vi "PFI-28000-Chan-Bridge_Get Filter Cutoff.vi"(8 "error in (no error)":errorcluster, 11 "PFI-28000-Chan-Bridge in":refnum<class "PFI-28000-Chan-Bridge.lvclass">) -> (0 "error out":errorcluster, 2 "Filter Cutoff":dbl, 3 "PFI-28000-Chan-Bridge out":refnum<class "PFI-28000-Chan-Bridge.lvclass">)   [LabVIEW 2017, in "PFI-28000-Chan-Bridge.lvclass"]
uses:
  PFI-28000-Chan-Bridge.lvclass
  C:/wc/07143 Precision Filters 28000 Support/Driver/source/Channel/PFI-28000-Channel.lvclass
  Utilities/PFI-28000-Utils.lvlib
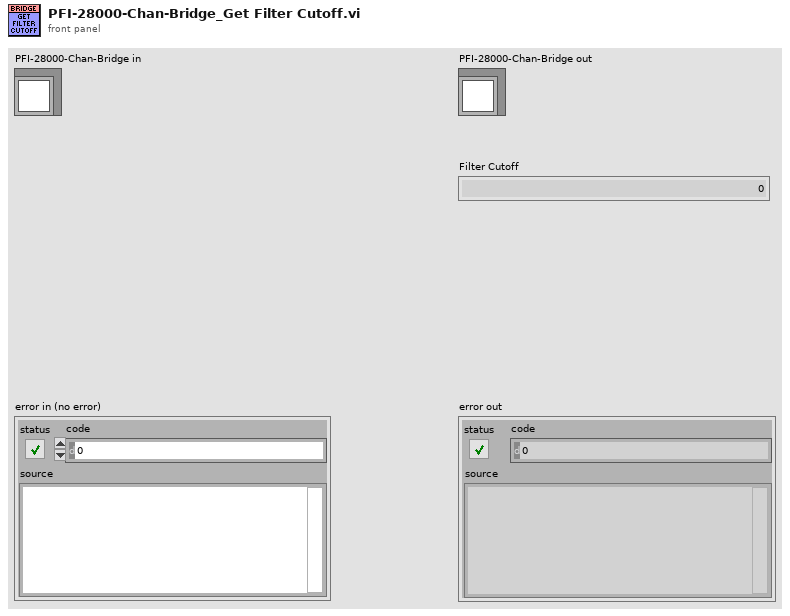
[diagram p1: front panel]
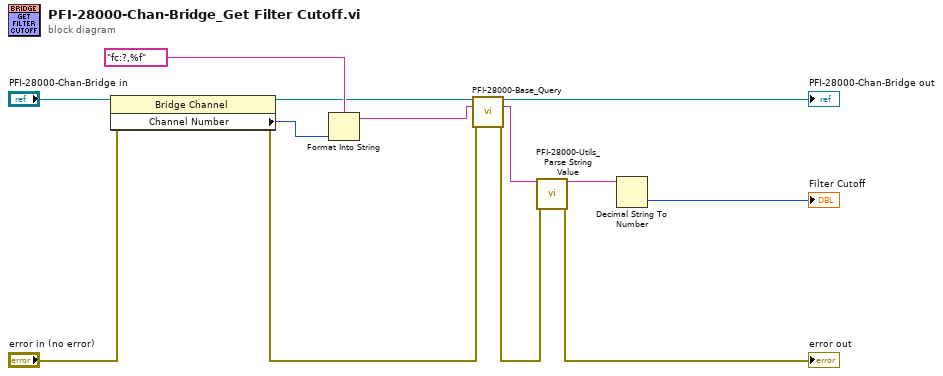
[diagram p0: block diagram]
diagram:
  n1 = property class="Bridge Channel"(reference="PFI-28000-Chan-Bridge in", error in="error in (no error)") -> (reference out=w9:refnum<class "PFI-28000-Chan-Bridge.lvclass">, error out=w6:errorcluster, "Channel Number"=w11:i32)
  n2 = Format Into String(format string="fc:?,%f" ("empty string"), w11) -> (resulting string=w7:string)  [unwired: 2 in, 1 out]
  n3 = call-dynamic "PFI-28000-Base_Query.vi"("PFI-28000-Base in"=w9, "Command"=w7, "error in (no error)"=w6) -> ("PFI-28000-Base out"=→"PFI-28000-Chan-Bridge out":refnum<class "PFI-28000-Chan-Bridge.lvclass">, "Response"=w3:string, "error out"=w5:errorcluster)  [unwired: 9 in, 1 out]
  n4 = call "PFI-28000-Utils_Parse String Value.vi"("String"=w3, "error in (no error)"=w5) -> ("String Value"=w2:string, "error out"=→"error out":errorcluster)  [unwired: 11 in, 1 out]
  n5 = Decimal String To Number(string=w2) -> (number=→"Filter Cutoff":i32)  [unwired: 2 in, 1 out]
